vi "Test Limits.vi"(0 "Config In":T2={"DAQ Settings"={"Trigger Type"=enum."Manual", "Trigger Samples"=0, "Pretrigger Samples"=0, "Trigger Interval"=0.0, "Time Units"=FALSE, "Auto Save"=FALSE, "Sample Rate"=7.0, "Select Analog"=FALSE, "Trigger Value"=0.0, "Trigger Stop Method"=enum."Use Samples Value to Stop Trigger", "Rate Sec/Min"=FALSE, "Save Mode"=enum."Single File", "File Size Limit"=0.0, "Log File Type"=enum."Basic", "Trigger Data Index"=0}, "Channels"=[], "Header"={"TA Number"="", "Test Name"="", "Serial Number"="", "Technician"=""}, "Graph Settings"={"Graph Labels"=[], [], [], [], [], [], [], [], [], [], [], [], [], "Graph Toggles"=[], "Axis Toggles"=[], "Graph Range"=enum."1"}, "Test Limits"=[], "All Type Info"=[], "Save Mode"=enum."Single File"} {"DAQ Settings"."Trigger Interval" min=0.0; "DAQ Settings"."Pretrigger Samples" min=0; "DAQ Settings"."Trigger Samples" min=0}, 5 "Channel Select":i32, 7 "Sensors":T1(array[cluster])) -> (4 "Config Out":T2={"DAQ Settings"={"Trigger Type"=enum."Manual", "Trigger Samples"=0, "Pretrigger Samples"=0, "Trigger Interval"=0.0, "Time Units"=FALSE, "Auto Save"=FALSE, "Sample Rate"=7.0, "Select Analog"=FALSE, "Trigger Value"=0.0, "Trigger Stop Method"=enum."Use Samples Value to Stop Trigger", "Rate Sec/Min"=FALSE, "Save Mode"=enum."Single File", "File Size Limit"=0.0, "Log File Type"=enum."Basic", "Trigger Data Index"=0}, "Channels"=[], "Header"={"TA Number"="", "Test Name"="", "Serial Number"="", "Technician"=""}, "Graph Settings"={"Graph Labels"=[], [], [], [], [], [], [], [], [], [], [], [], [], "Graph Toggles"=[], "Axis Toggles"=[], "Graph Range"=enum."1"}, "Test Limits"=[], "All Type Info"=[], "Save Mode"=enum."Single File"} {"DAQ Settings"."Trigger Interval" min=0.0; "DAQ Settings"."Pretrigger Samples" min=0; "DAQ Settings"."Trigger Samples" min=0})   [LabVIEW 2019]
uses:
  Type Defs and Controls/Sensor Config.ctl
  Type Defs and Controls/DAQ Settings.ctl
  Type Defs and Controls/Trigger Stop Method.ctl
  Type Defs and Controls/Log File Type.ctl
  Type Defs and Controls/Channel Config.ctl
  Type Defs and Controls/Header.ctl
  Type Defs and Controls/Graph Settings Type Def.ctl
  Type Defs and Controls/Test Limits.ctl
  Type Defs and Controls/All Part Info.ctl
  Type Defs and Controls/Part Info.ctl
panel:
  in  "EU High Min":dbl format="%.3f Volts"
  in  "EU High Max":dbl format="%.3f Volts"
  out "Acquire":bool
  in  "Pk-Pk Minimum":dbl format="%.3f Volts"
  in  "Pk-Pk Maximum":dbl format="%.3f Volts"
  in  "Enable Limits":bool
  in  "RMS Minimum":dbl format="%.3f Volts"
  in  "RMS Maximum":dbl format="%.3f Volts"
  in  "Enable Limits":bool
  in  "Freq Minimum":dbl format="%.1f Hz"
  in  "Freq Maximum":dbl format="%.1f Hz"
  in  "Enable Limits":bool
  in  "EU Low Min":dbl format="%.3f Volts"
  in  "EU Low Max":dbl format="%.3f Volts"
  in  "Cancel":bool
  in  "OK":bool
  out "Name":string
  # "EU Limits"
  # "RMS Limits"
  # "Pk-Pk Limits"
  # "Frequency Limits"
  # "All Signals that have matching High and Low Limits will not be in Functional data file."
  # "EGU"
  # "EGU"
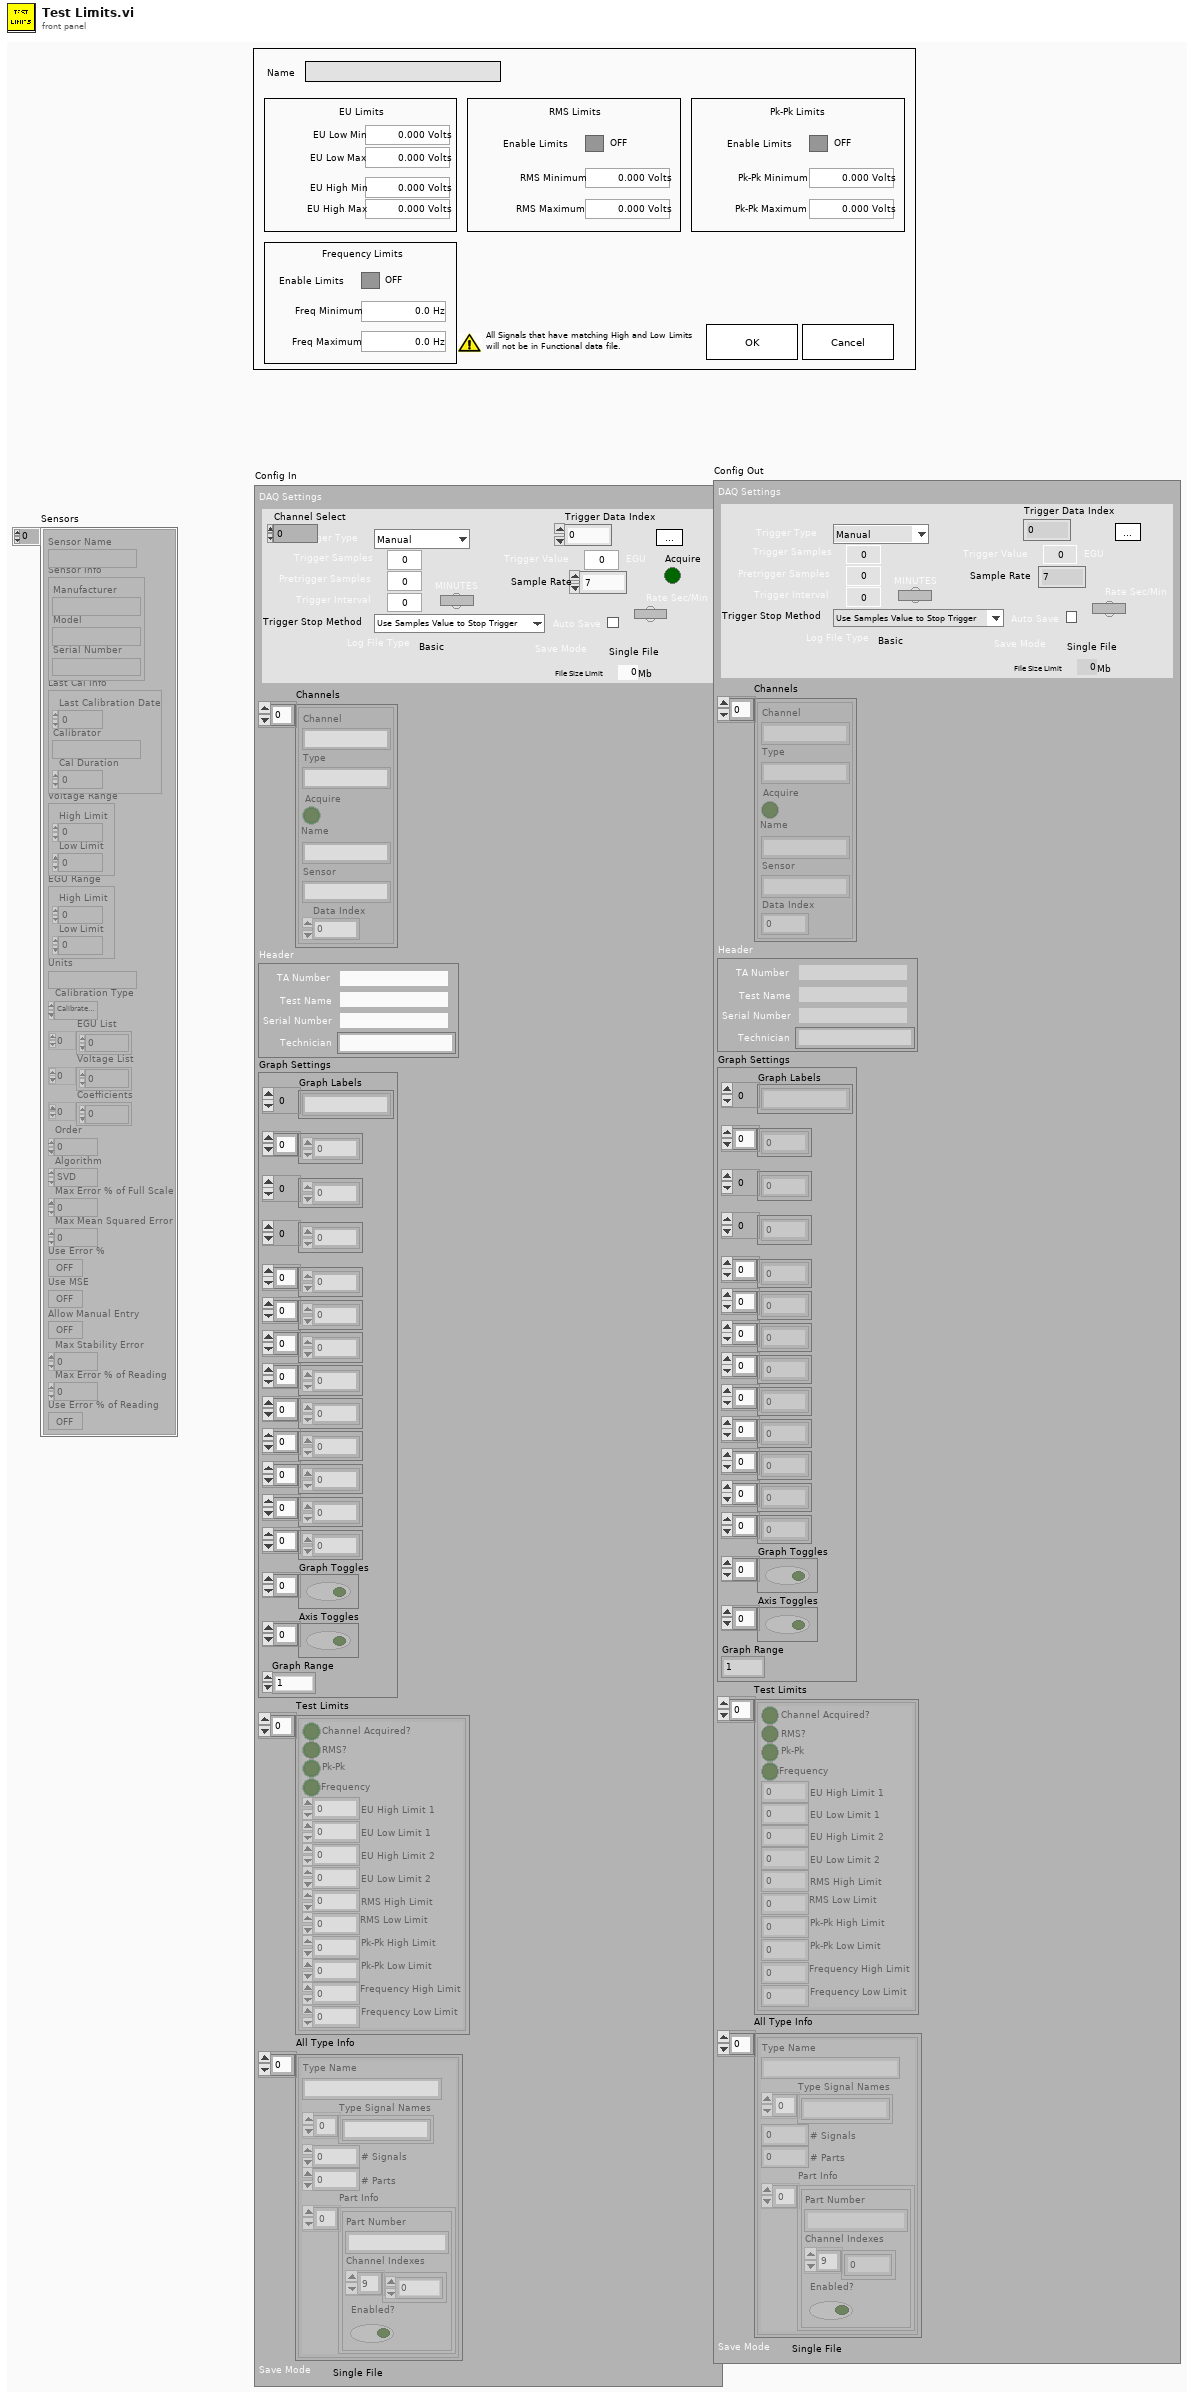
[diagram p1: front panel]
types:
  T1 = cluster{"Sensor Name":string, "Sensor Info":cluster{"Manufacturer":string, "Model":string, "Serial Number":string}, "Last Cal Info":cluster{"Last Calibration Date":dbl, "Calibrator":string, "Cal Duration":i32}, "Voltage Range":cluster{"High Limit":dbl, "Low Limit":dbl}, "EGU Range":cluster{"High Limit":dbl, "Low Limit":dbl}, "Units":string, "Calibration Type":enum16{"Calibrate Analog", "Compare Analog Calibration"}, "EGU List":dbl[], "Voltage List":dbl[], "Coefficients":dbl[], "Order":i32, "Algorithm":enum32{"SVD", "Givens", "Givens2", "Householder", "LU Decomposition", "Cholesky"}, "Max Error % of Full Scale":dbl, "Max Mean Squared Error":dbl, "Use Error %":bool, "Use MSE":bool, "Allow Manual Entry":bool, "Max Stability Error":dbl, "Max Error % of Reading":dbl, "Use Error % of Reading":bool}[]
  T2 = typedef "Sensor Config.ctl" = cluster{"DAQ Settings":T3, "Channels":T6[], "Header":T7, "Graph Settings":T8, "Test Limits":T9[], "All Type Info":T10, "Save Mode":enum16{"Single File", "Segmented Files", "New File at Midnight"}}
  T3 = typedef "DAQ Settings.ctl" = cluster{"Trigger Type":enum16{"Manual", "Timed", "Analog Rising", "Analog Falling"}, "Trigger Samples":i32, "Pretrigger Samples":i32, "Trigger Interval":dbl, "Time Units":bool, "Auto Save":bool, "Sample Rate":dbl, "Select Analog":bool, "Trigger Value":dbl, "Trigger Stop Method":T4, "Rate Sec/Min":bool, "Save Mode":enum16{"Single File", "Segmented Files", "New File at Midnight"}, "File Size Limit":dbl, "Log File Type":T5, "Trigger Data Index":u32}
  T4 = typedef "Trigger Stop Method.ctl" = enum16{"Use Samples Value to Stop Trigger", "Use Threshold to Stop Trigger"}
  T5 = typedef "Log File Type.ctl" = enum16{"Basic", "RTS"}
  T6 = typedef "Channel Config.ctl" = cluster{"Channel":string, "Type":string, "Acquire":bool, "Name":string, "Sensor":string, "Data Index":u32}
  T7 = typedef "Header.ctl" = cluster{"TA Number":string, "Test Name":string, "Serial Number":string, "Technician":string}
  T8 = typedef "Graph Settings Type Def.ctl" = cluster{"Graph Labels":string[], u8[], i16[], u32[], u8[], u8[], u8[], u32[], u8[], u8[], u8[], dbl[], dbl[], "Graph Toggles":bool[], "Axis Toggles":bool[], "Graph Range":enum16{"1", "2", "3", "4", "5", "10", "15", "30", "60"}}
  T9 = typedef "Test Limits.ctl" = cluster{"Channel Acquired?":bool, "RMS?":bool, "Pk-Pk":bool, "Frequency":bool, "EU High Limit 1":dbl, "EU Low Limit 1":dbl, "EU High Limit 2":dbl, "EU Low Limit 2":dbl, "RMS High Limit":dbl, "RMS Low Limit":dbl, "Pk-Pk High Limit ":dbl, "Pk-Pk Low Limit":dbl, "Frequency High Limit":dbl, "Frequency Low Limit":dbl}
  T10 = typedef "All Part Info.ctl" = cluster{"Type Name":string, "Type Signal Names":string[], "# Signals":i32, "# Parts":i32, "Part Info":T11[]}[]
  T11 = typedef "Part Info.ctl" = cluster{"Part Number":string, "Channel Indexes":u16[], "Enabled?":bool}
  T12 = cluster{"Sensor Name":string, "Sensor Info":cluster{"Manufacturer":string, "Model":string, "Serial Number":string}, "Last Cal Info":cluster{"Last Calibration Date":dbl, "Calibrator":string, "Cal Duration":i32}, "Voltage Range":cluster{"High Limit":dbl, "Low Limit":dbl}, "EGU Range":cluster{"High Limit":dbl, "Low Limit":dbl}, "Units":string, "Calibration Type":enum16{"Calibrate Analog", "Compare Analog Calibration"}, "EGU List":dbl[], "Voltage List":dbl[], "Coefficients":dbl[], "Order":i32, "Algorithm":enum32{"SVD", "Givens", "Givens2", "Householder", "LU Decomposition", "Cholesky"}, "Max Error % of Full Scale":dbl, "Max Mean Squared Error":dbl, "Use Error %":bool, "Use MSE":bool, "Allow Manual Entry":bool, "Max Stability Error":dbl, "Max Error % of Reading":dbl, "Use Error % of Reading":bool}
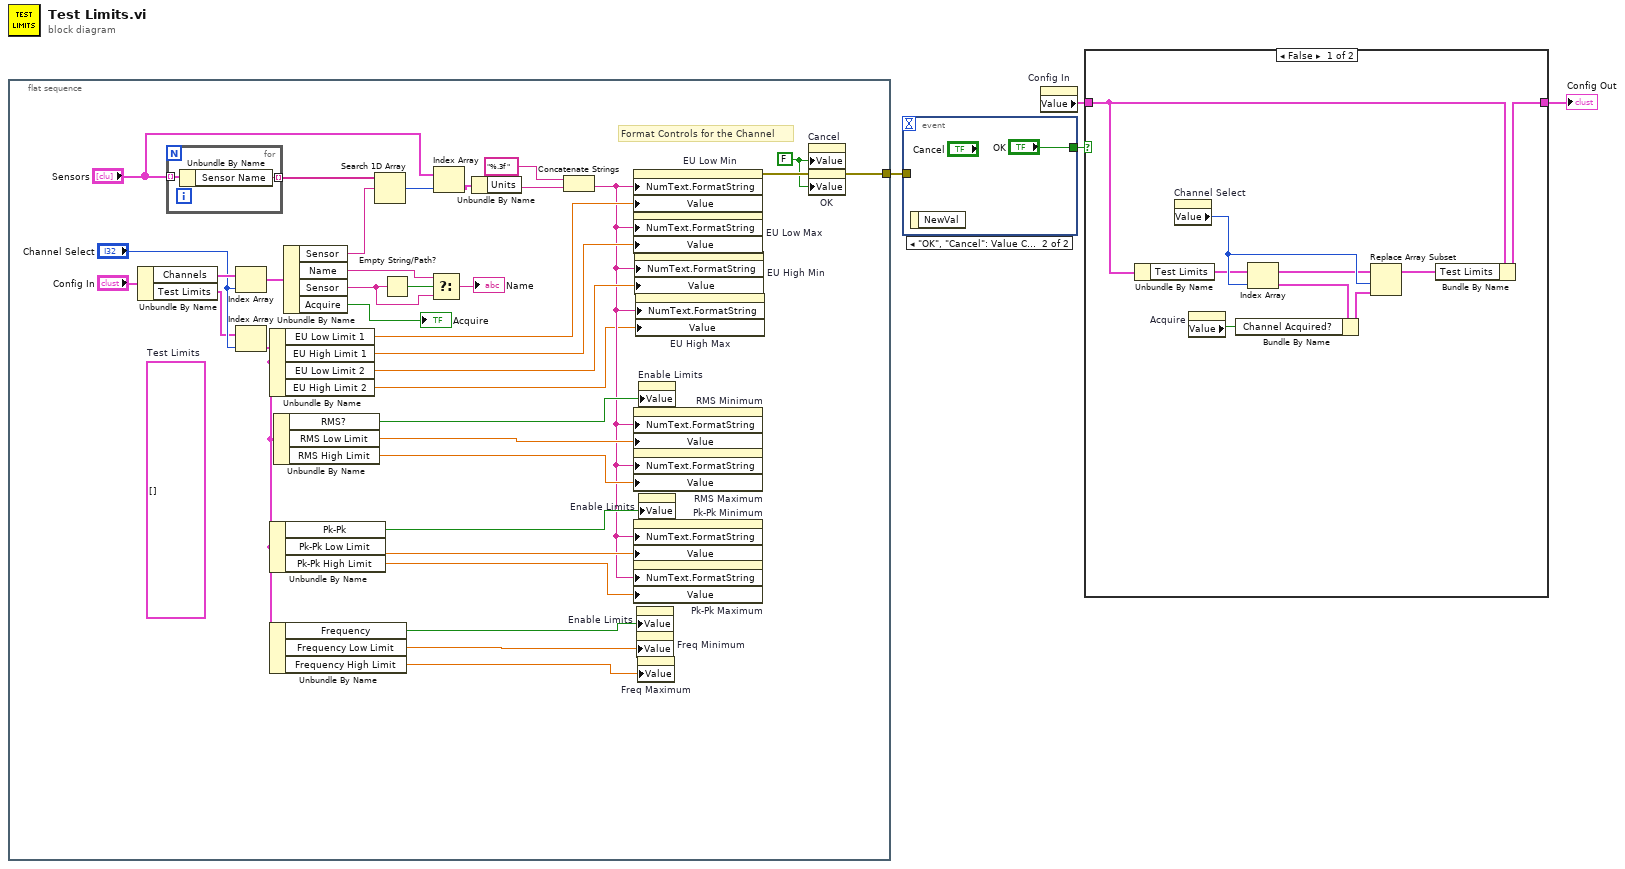
[diagram p0: block diagram]
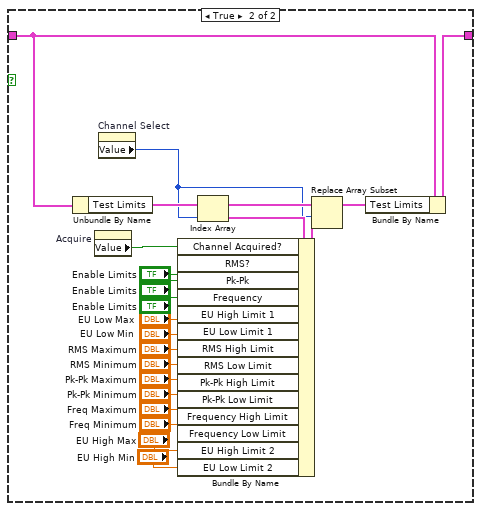
[diagram p2: hidden frame]
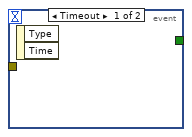
[diagram p3: hidden frame]
diagram:
  n1 = flat-sequence {
    tunnel: [w15] -> w4
    frame #0 {
      (unwired) T9[] []  # Test Limits
      w13 = FALSE ("Cancel")
      # "Format Controls for the Channel"
      n2 = Unbundle By Name("Config In") -> ("Channels"=w38:T6[], "Test Limits"=w28:T9[])
      n3 = for {
        tunnel: "Sensors" -> [w41] mode=indexing
        tunnel: [w40] -> w36 mode=indexing
        n4 = Unbundle By Name(w41) -> ("Sensor Name"=w40:string)
      }
      n5 = Index Array(array=w38, index="Channel Select") -> (element=w37:T6)
      n6 = Index Array(array=w28, index="Channel Select") -> (element=w19:T9)
      n7 = Unbundle By Name(w19) -> ("EU Low Limit 1"=w27:dbl, "EU High Limit 1"=w26:dbl, "EU Low Limit 2"=w7:dbl, "EU High Limit 2"=w5:dbl)
      n8 = Unbundle By Name(w19) -> ("Pk-Pk"=w17:bool, "Pk-Pk Low Limit"=w23:dbl, "Pk-Pk High Limit"=w22:dbl)
      n9 = Unbundle By Name(w19) -> ("Frequency"=w16:bool, "Frequency Low Limit"=w21:dbl, "Frequency High Limit"=w20:dbl)
      n10 = Unbundle By Name(w19) -> ("RMS?"=w18:bool, "RMS Low Limit"=w25:dbl, "RMS High Limit"=w24:dbl)
      n11 = Unbundle By Name(w37) -> ("Sensor"=w35:string, "Name"=w10:string, "Sensor"=w9:string, "Acquire"=→"Acquire":bool)
      n12 = Search 1D Array(1D array=w36, element=w35) -> (index of element=w34:i32)  [unwired: 1 in]
      n13 = Empty String/Path?(string/path=w9) -> (empty?=w11:bool)
      n14 = Select(t=w10, s=w11, f=w9) -> (s? t:f=→"Name":string)
      n15 = Index Array(array="Sensors", index=w34) -> (element=w32:T12)
      n16 = Unbundle By Name(w32) -> ("Units"=w31:string)
      n17 = Concatenate Strings("%.3f " ("string"), w31) -> (w6:string)
      n18 = property on="EU Low Min" class="DigNum (strict)"("NumText.FormatString"=w6, "Value"=w27) -> (error out=w14:errorcluster)  [unwired: 2 in, 1 out]
      n19 = property on="EU Low Max" class="DigNum (strict)"("NumText.FormatString"=w6, "Value"=w26) -> ()  [unwired: 2 in, 2 out]
      n20 = property on="RMS Minimum" class="DigNum (strict)"("NumText.FormatString"=w6, "Value"=w25) -> ()  [unwired: 2 in, 2 out]
      n21 = property on="RMS Maximum" class="DigNum (strict)"("NumText.FormatString"=w6, "Value"=w24) -> ()  [unwired: 2 in, 2 out]
      n22 = property on="Pk-Pk Minimum" class="DigNum (strict)"("NumText.FormatString"=w6, "Value"=w23) -> ()  [unwired: 2 in, 2 out]
      n23 = property on="Pk-Pk Maximum" class="DigNum (strict)"("NumText.FormatString"=w6, "Value"=w22) -> ()  [unwired: 2 in, 2 out]
      n24 = property on="EU High Min" class="DigNum (strict)"("NumText.FormatString"=w6, "Value"=w7) -> ()  [unwired: 2 in, 2 out]
      n25 = property on="EU High Max" class="DigNum (strict)"("NumText.FormatString"=w6, "Value"=w5) -> ()  [unwired: 2 in, 2 out]
      n26 = property on="Enable Limits" class="Bool (strict)"("Value"=w16) -> ()  [unwired: 2 in, 2 out]
      n27 = property on="Freq Minimum" class="DigNum (strict)"("Value"=w21) -> ()  [unwired: 2 in, 2 out]
      n28 = property on="Freq Maximum" class="DigNum (strict)"("Value"=w20) -> ()  [unwired: 2 in, 2 out]
      n29 = property on="Enable Limits" class="Bool (strict)"("Value"=w18) -> ()  [unwired: 2 in, 2 out]
      n30 = property on="Enable Limits" class="Bool (strict)"("Value"=w17) -> ()  [unwired: 2 in, 2 out]
      n31 = property on="Cancel" class="Bool (strict)"("Value"=w13) -> ()  [unwired: 2 in, 2 out]
      n32 = property on="OK" class="Bool (strict)"(error in=w14, "Value"=w13) -> (error out=w15:errorcluster)  [unwired: 1 in, 1 out]
    }
  }
  n33 = event shown="[1] \"OK\", \"Cancel\": Value Change" {
    selector: _ -> [_ _]
    dyn-events: _ -> [_ _]
    timeout: _ -> [_ _]
    tunnel: [_ "OK"] -> w3
    tunnel: w4 -> [_ _]
    event Timeout {
      (unwired) FALSE
      n34 = event-data() -> ()  [unwired: 1 in, 2 out]
    }
    event "OK", "Cancel": Value Change {
      n35 = event-data() -> ()  [unwired: 1 in, 1 out]
    }
  }
  n36 = property on="Config In" class="Clust (strict)"() -> ("Value"=w2:T2)  [unwired: 2 in, 2 out]
  n37 = case shown="False" w3 {
    tunnel: w2 -> [w49 w70]
    tunnel: [w50 w71] -> w1
    frame False {
      n38 = Unbundle By Name(w49) -> ("Test Limits"=w44:T9[])
      n39 = property on="Channel Select" class="DigNum (strict)"() -> ("Value"=w45:i32)  [unwired: 2 in, 2 out]
      n40 = property on="Acquire" class="Bool (strict)"() -> ("Value"=w47:bool)  [unwired: 2 in, 2 out]
      n41 = Index Array(array=w44, index=w45) -> (element=w48:T9)
      n42 = Bundle By Name(cluster=w48, "Channel Acquired?"=w47) -> (w46:T9)
      n43 = Replace Array Subset(array=w44, new element=w46, index=w45) -> (w43:T9[])
      n44 = Bundle By Name(cluster=w49, "Test Limits"=w43) -> (w50:T2)
    }
    frame True {
      n45 = Unbundle By Name(w70) -> ("Test Limits"=w55:T9[])
      n46 = property on="Acquire" class="Bool (strict)"() -> ("Value"=w68:bool)  [unwired: 2 in, 2 out]
      n47 = property on="Channel Select" class="DigNum (strict)"() -> ("Value"=w54:i32)  [unwired: 2 in, 2 out]
      n48 = Index Array(array=w55, index=w54) -> (element=w69:T9)
      n49 = Bundle By Name(cluster=w69, "Channel Acquired?"=w68, "RMS?"="Enable Limits", "Pk-Pk"="Enable Limits", "Frequency"="Enable Limits", "EU High Limit 1"="EU Low Max", "EU Low Limit 1"="EU Low Min", "RMS High Limit"="RMS Maximum", "RMS Low Limit"="RMS Minimum", "Pk-Pk High Limit"="Pk-Pk Maximum", "Pk-Pk Low Limit"="Pk-Pk Minimum", "Frequency High Limit"="Freq Maximum", "Frequency Low Limit"="Freq Minimum", "EU High Limit 2"="EU High Max", "EU Low Limit 2"="EU High Min") -> (w67:T9)
      n50 = Replace Array Subset(array=w55, new element=w67, index=w54) -> (w53:T9[])
      n51 = Bundle By Name(cluster=w70, "Test Limits"=w53) -> (w71:T2)
    }
  }
  "Config Out" <- w1
